vi "Test Get Child Classes.vi"() -> ()   [LabVIEW 2018]
uses:
  Plugins/Utility/Test Classes/String/String.lvclass
  C:/Users/UKHornP/Documents/Work/Projects/Assert_API/Plugins/Utility/Test Classes/Test.lvclass
  Plugins/Utility/Test Classes/Integer/Integer.lvclass
  Plugins/Utility/Test Classes/Floating Point/Floating Point.lvclass
  Plugins/Utility/Test Classes/Boolean/Boolean.lvclass
  Plugins/Utility/Test Classes/Test.lvclass
panel:
  out "Array":string[](array[string])
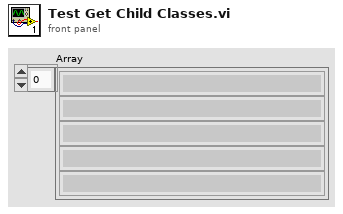
[diagram p1: front panel]
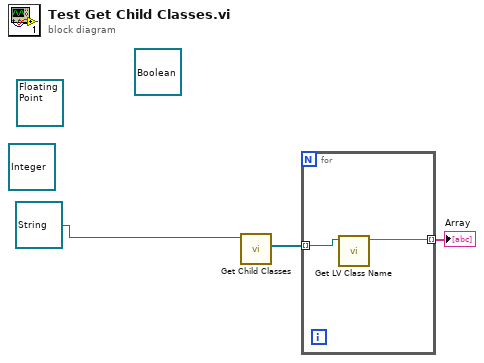
[diagram p0: block diagram]
diagram:
  (unwired) refnum<class "Boolean.lvclass"> refnum ("Boolean.lvclass")
  (unwired) refnum<class "Floating Point.lvclass"> refnum ("Floating Point.lvclass")
  (unwired) refnum<class "Integer.lvclass"> refnum ("Integer.lvclass")
  n1 = call "Get Child Classes.vi"("Test in"=refnum<class "String.lvclass"> refnum ("String.lvclass")) -> ("Child Classes"=w3:refnum<class "Test.lvclass">[])  [unwired: 9 in, 1 out]
  n2 = for {
    tunnel: w3 -> [w5] mode=indexing
    tunnel: [w4] -> w2 mode=indexing
    n3 = call <vilib>:"Get LV Class Name.vi"("object"=w5) -> ("class name"=w4:string)  [unwired: 9 in, 1 out]
  }
  "Array" <- w2
